vi "command_code_type.vi"(11 "Line in":string) -> (2 "Code type out":T1, 3 "Line out":string)   [LabVIEW 2017, in "labview-standard-library.lvlib"]
uses:
  labview-standard-library.lvlib
  type-defs/code_types.ctl
panel:
  in  "code types":T1
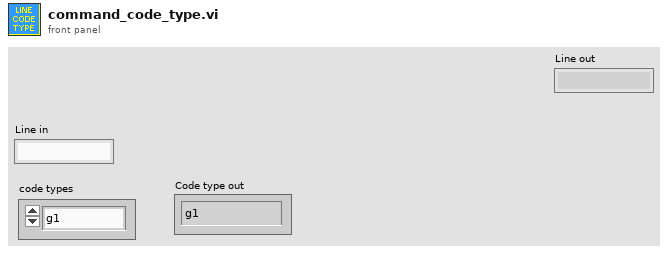
[diagram p1: front panel]
types:
  T1 = typedef "labview-standard-library.lvlib/code_types.ctl" = enum16{"g1", "g2", "g3", "g4", "g7", "m0", "m2", "t0", "t1", "t2", "comment"}
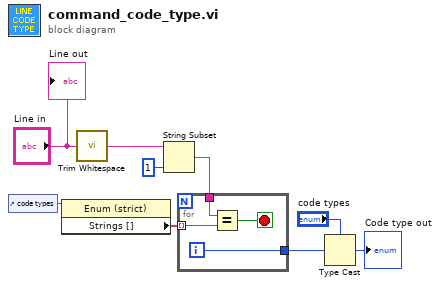
[diagram p0: block diagram]
diagram:
  n1 = control-ref of="code types"() -> (w4:refnum<vi>)
  n2 = property class="Enum (strict)"(reference=w4) -> ("Strings []"=w3:string[])  [unwired: 1 in, 2 out]
  n3 = call <vilib>:"Trim Whitespace.vi"("string"="Line in") -> ("trimmed string"=w1:string)  [unwired: 1 in]
  n4 = String Subset(string=w1, length (rest)=1 ("length (rest)")) -> (substring=w7:string)  [unwired: 1 in]
  n5 = for {
    tunnel: w3 -> [w13] mode=indexing
    tunnel: w7 -> [w12]
    tunnel: [w10] -> w8
    i -> [w10]
    stop <- w11 stop-if-true
    n6 = Equal?(x=w12, y=w13) -> (x = y?=w11:bool)
  }
  n7 = Type Cast(type="code types", x=w8) -> (*(type *) &x=→"Code type out":T1)
  "Line out" <- "Line in"
